vi "Framework_Initialize.vi"(8 "error in (no error)":errorcluster, 11 "AB_PackedLibrary in":refnum<class "AB_PackedLibrary.lvclass">) -> (0 "error out":errorcluster, 1 "helpTopics":string[](array[string]), 2 "pageTitles":string[](array[string]), 3 "AB_PackedLibrary out":refnum<class "AB_PackedLibrary.lvclass">, 4 "helpFile":string, 5 "pages":path[](array[path]))   [LabVIEW 2020, in "AB_PackedLibrary.lvclass"]
uses:
  <vilib>/AppBuilder/AB_Classes/PackedLib/AB_PackedLibrary.lvclass
panel:
  in  "pageTitles_DLL":string[](array[string])=["Information", "Source Files", "Destinations", "Source File Settings", "Advanced", "Additional Exclusions", "Connector Pane State", "Version Information", "Pre/Post Build Actions", "Preview"]
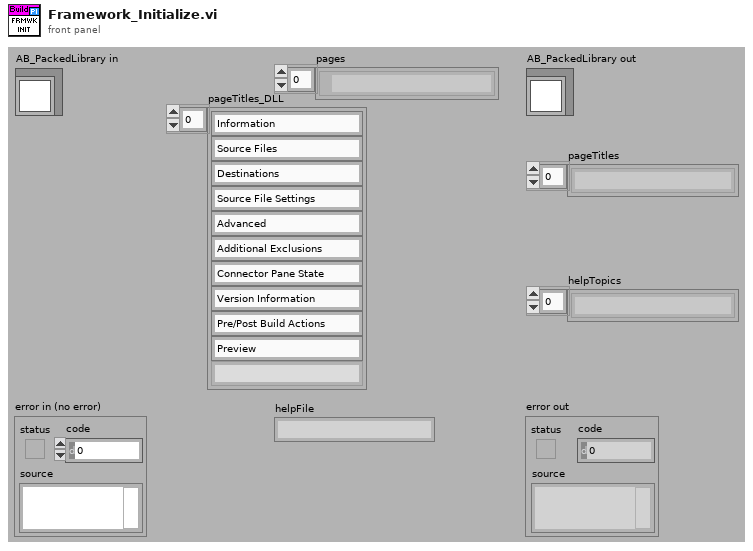
[diagram p1: front panel]
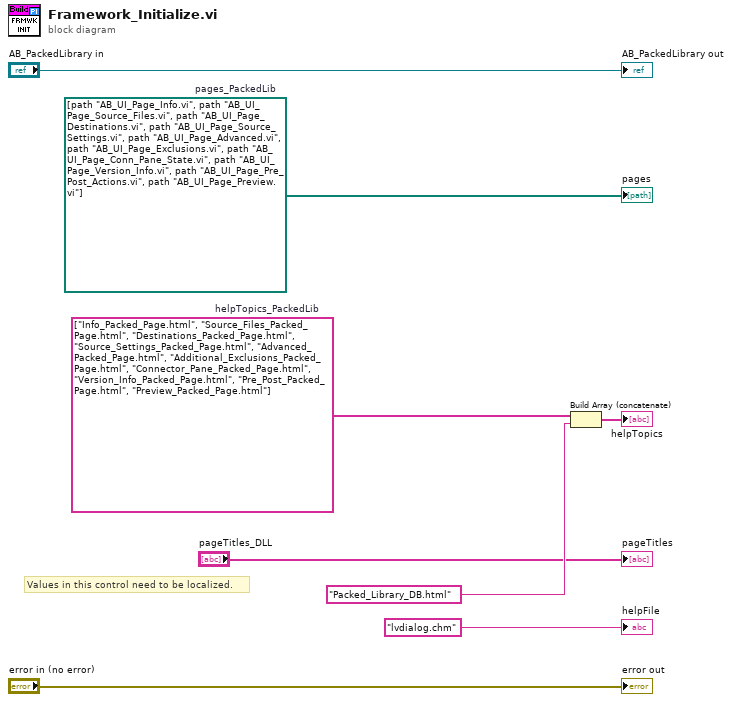
[diagram p0: block diagram]
diagram:
  w2 = string[] ["Info_Packed_Page.html", "Source_Files_Packed_Page.html", "Destinations_Packed_Page.html", "Source_Settings_Packed_Page.html", "Advanced_Packed_Page.html", "Additional_Exclusions_Packed_Page.html", "Connector_Pane_Packed_Page.html", "Version_Info_Packed_Page.html", "Pre_Post_Packed_Page.html", "Preview_Packed_Page.html"]  # helpTopics_PackedLib
  w3 = path[] [path "AB_UI_Page_Info.vi", path "AB_UI_Page_Source_Files.vi", path "AB_UI_Page_Destinations.vi", path "AB_UI_Page_Source_Settings.vi", path "AB_UI_Page_Advanced.vi", path "AB_UI_Page_Exclusions.vi", path "AB_UI_Page_Conn_Pane_State.vi", path "AB_UI_Page_Version_Info.vi", path "AB_UI_Page_Pre_Post_Actions.vi", path "AB_UI_Page_Preview.vi"]  # pages_PackedLib
  # "Values in this control need to be localized."
  n1 = Build Array (concatenate)(w2, "Packed_Library_DB.html" ("HTML filename")) -> (→"helpTopics":string[])
  "error out" <- "error in (no error)"
  "AB_PackedLibrary out" <- "AB_PackedLibrary in"
  "pages" <- w3
  "pageTitles" <- "pageTitles_DLL"
  "helpFile" <- "lvdialog.chm" ("CHM or HLP filename (lvdialog.chm)")
